vi "Class Reference FGV.vi"(7 "Options":T2, 8 "error in":errorcluster, 11 "Class Cluster In":T1) -> (0 "error out":errorcluster, 3 "Class Cluster Out":T1)   [LabVIEW 2023, in "HardwareAbstractionLayer_LVOOP.lvlib" / "Main.lvclass"]
uses:
  Main.lvclass
  Class Options.ctl
  Class Ref.ctl
  DMM/DMM.lvclass
  Function Generator/Function Generator.lvclass
  Oscilloscope/Oscilloscope.lvclass
  PowerSupply/PowerSupply.lvclass
  Teststand/Teststand.lvclass
  Analog Output/AO/AO.lvclass
  Analog Input/AI/AI.lvclass
  Database/Database.lvclass
  Digital Output/DO_class/DO.lvclass
  Digital Input/DI_class/DI.lvclass
  PWM Output/PWM Output_class/PWM Output.lvclass
  PWM Input/PWM Input_class/PWM Input.lvclass
  NI Switch/NISwitch_class/NISwitch.lvclass
  Modbus/Modbus_class/Modbus.lvclass
  CAN/CAN Lib/CAN_class/CAN.lvclass
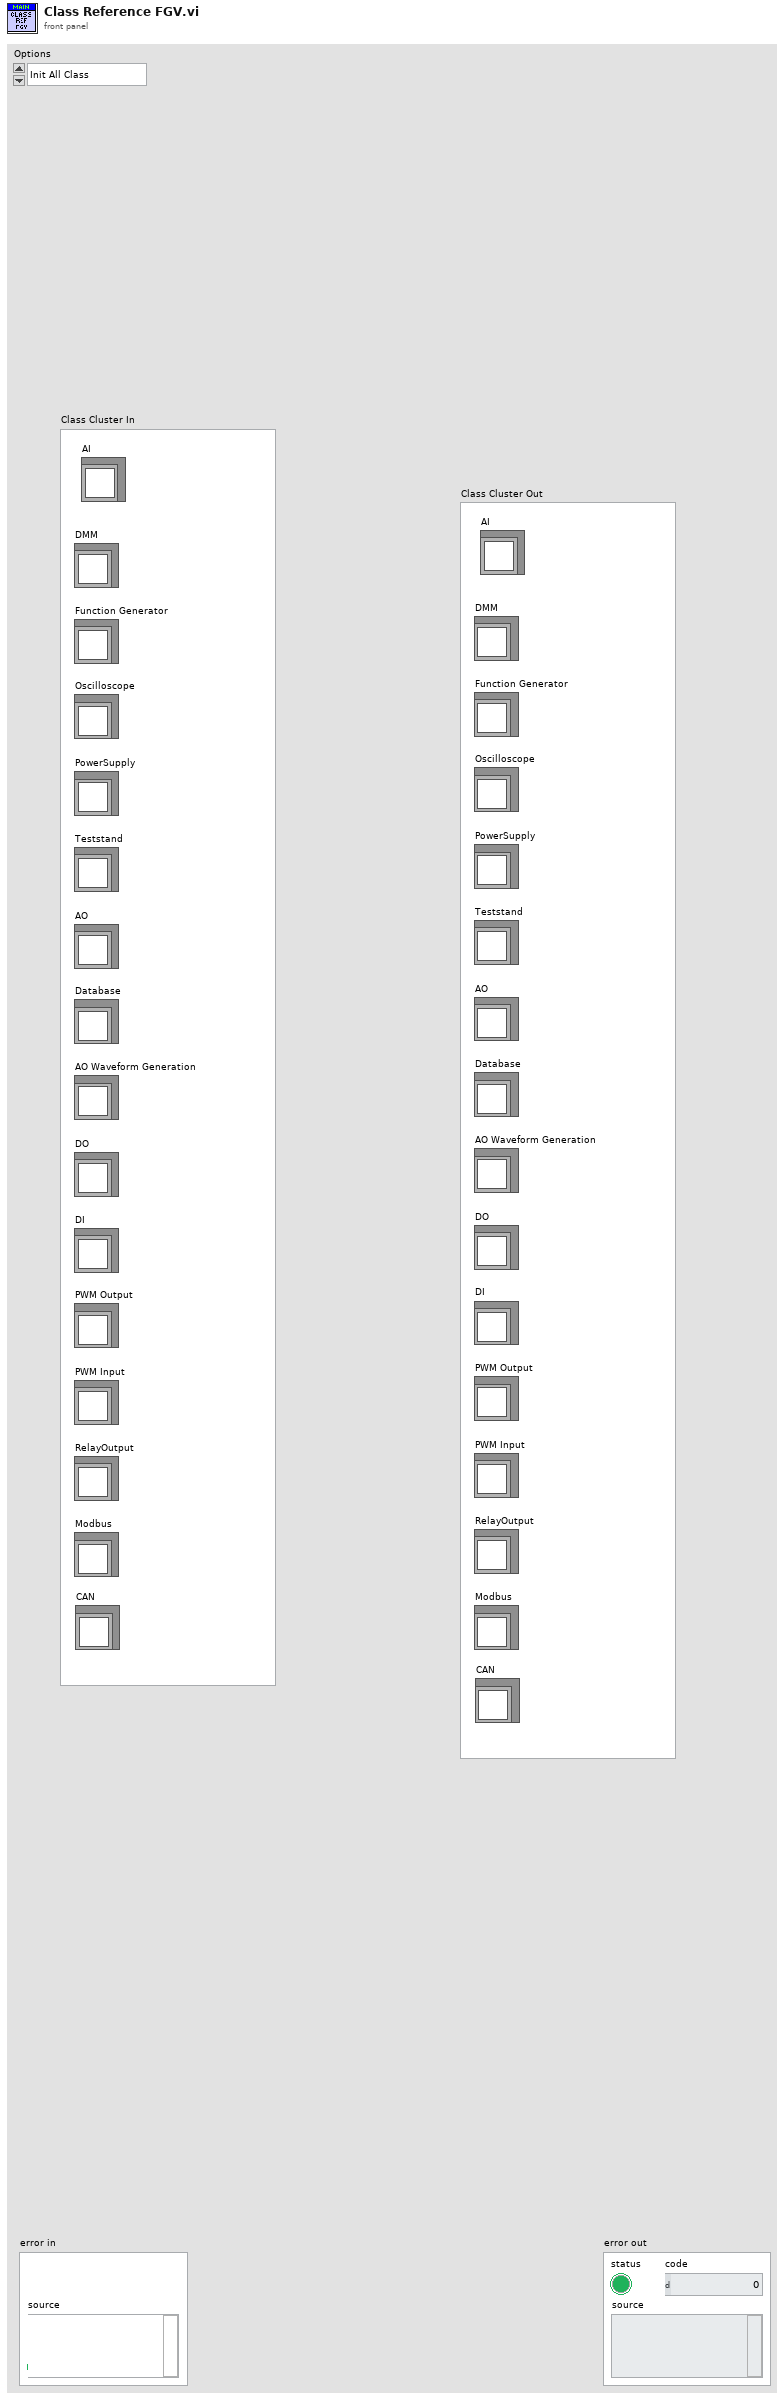
[diagram p1: front panel]
types:
  T1 = typedef "HardwareAbstractionLayer_LVOOP.lvlib/Main.lvclass/Class Ref.ctl" = cluster{"DMM":refnum<class "DMM.lvclass">, "Function Generator":refnum<class "Function Generator.lvclass">, "Oscilloscope":refnum<class "Oscilloscope.lvclass">, "PowerSupply":refnum<class "PowerSupply.lvclass">, "Teststand":refnum<class "Teststand.lvclass">, "AO":refnum<class "AO.lvclass">, "AI":refnum<class "AI.lvclass">, "Database":refnum<class "Database.lvclass">, "AO Waveform Generation":refnum<class "AO.lvclass">, "DO":refnum<class "DO.lvclass">, "DI":refnum<class "DI.lvclass">, "PWM Output":refnum<class "PWM Output.lvclass">, "PWM Input":refnum<class "PWM Input.lvclass">, "RelayOutput":refnum<class "NISwitch.lvclass">, "Modbus":refnum<class "Modbus.lvclass">, "CAN":refnum<class "CAN.lvclass">}
  T2 = typedef "HardwareAbstractionLayer_LVOOP.lvlib/Main.lvclass/Class Options.ctl" = enum16{"Init All Class", "Read All Class", "Write AI Class", "Write AO Class", "Write AO Waveform Generation", "Write DI Class", "Write DO Class", "Write PWM Input Class", "Write PWM Output Class", "Exit"}
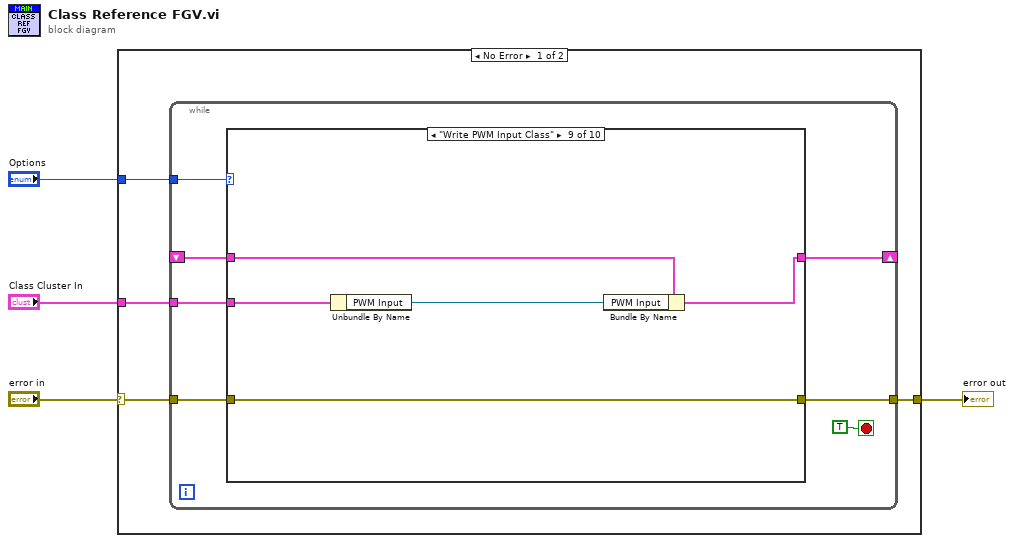
[diagram p0: block diagram]
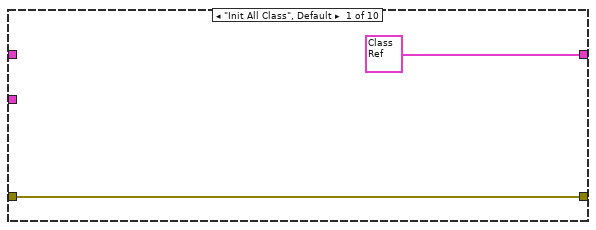
[diagram p2: hidden frame]
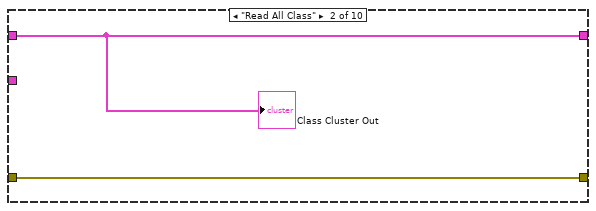
[diagram p3: hidden frame]
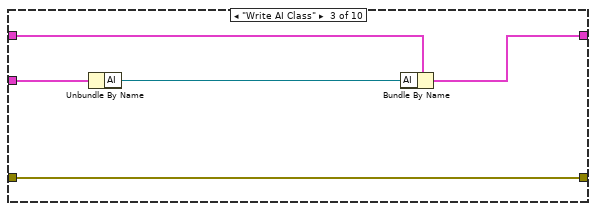
[diagram p4: hidden frame]
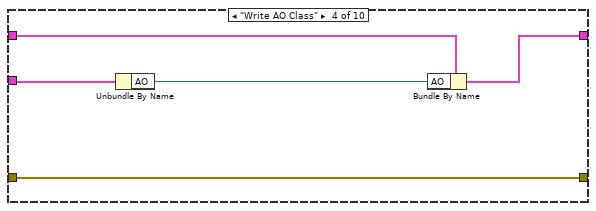
[diagram p5: hidden frame]
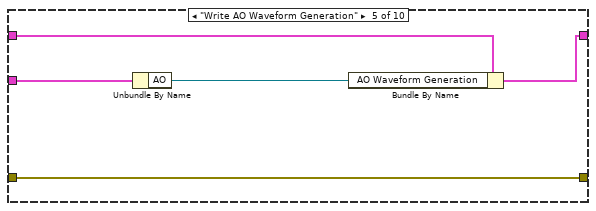
[diagram p6: hidden frame]
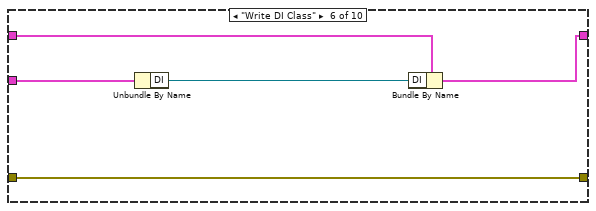
[diagram p7: hidden frame]
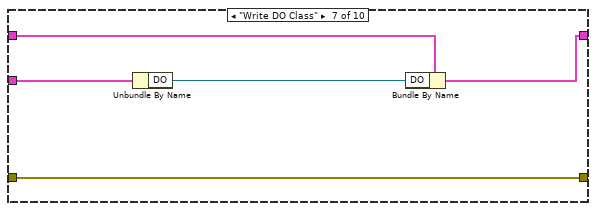
[diagram p8: hidden frame]
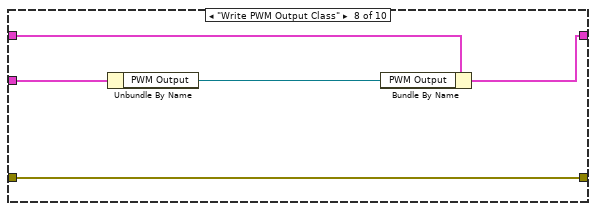
[diagram p9: hidden frame]
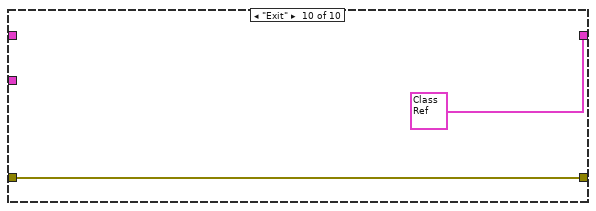
[diagram p10: hidden frame]
diagram:
  n1 = case shown="No Error" "error in" {
    selector: "error in" -> [w6 w57]
    tunnel: "Options" -> [w8 _]
    tunnel: "Class Cluster In" -> [w7 _]
    tunnel: [w5 w57] -> w1
    frame No Error {
      n2 = while {
        tunnel: w8 -> [w14]
        shift-right: [w12] -> _
        shift-left: _ -> [w13]
        tunnel: w7 -> [w11]
        tunnel: w6 -> [w10]
        tunnel: [w9] -> w5
        stop <- TRUE stop-if-true
        n3 = case shown="\"Write PWM Input Class\"" w14 {
          tunnel: w13 -> [_ w19 w23 w27 w32 w37 w42 w47 w52 _]
          tunnel: [T1 {"DMM"=refnum, "Function Generator"=refnum, "Oscilloscope"=refnum, "PowerSupply"=refnum, "Teststand"=refnum, "AO"=refnum, "AI"=refnum, "Database"=refnum, "AO Waveform Generation"=refnum, "DO"=refnum, "DI"=refnum, "PWM Output"=refnum, "PWM Input"=refnum, "RelayOutput"=refnum, "Modbus"=refnum, "CAN"=refnum} ("Class Cluster In") w19 w22 w26 w31 w36 w41 w46 w51 T1 {"DMM"=refnum, "Function Generator"=refnum, "Oscilloscope"=refnum, "PowerSupply"=refnum, "Teststand"=refnum, "AO"=refnum, "AI"=refnum, "Database"=refnum, "AO Waveform Generation"=refnum, "DO"=refnum, "DI"=refnum, "PWM Output"=refnum, "PWM Input"=refnum, "RelayOutput"=refnum, "Modbus"=refnum, "CAN"=refnum} ("Class Cluster In")] -> w12
          tunnel: w11 -> [_ _ w21 w25 w30 w35 w40 w45 w50 _]
          tunnel: w10 -> [w16 w18 w24 w29 w34 w39 w44 w49 w54 w55]
          tunnel: [w16 w18 w24 w29 w34 w39 w44 w49 w54 w55] -> w9
          frame "Init All Class", Default {
          }
          frame "Read All Class" {
            "Class Cluster Out" <- w19
          }
          frame "Write AI Class" {
            n4 = Unbundle By Name(w21) -> ("AI"=w20:refnum<class "AI.lvclass">)
            n5 = Bundle By Name(cluster=w23, "AI"=w20) -> (w22:T1)
          }
          frame "Write AO Class" {
            n6 = Unbundle By Name(w25) -> ("AO"=w28:refnum<class "AO.lvclass">)
            n7 = Bundle By Name(cluster=w27, "AO"=w28) -> (w26:T1)
          }
          frame "Write AO Waveform Generation" {
            n8 = Unbundle By Name(w30) -> ("AO"=w33:refnum<class "AO.lvclass">)
            n9 = Bundle By Name(cluster=w32, "AO Waveform Generation"=w33) -> (w31:T1)
          }
          frame "Write DI Class" {
            n10 = Unbundle By Name(w35) -> ("DI"=w38:refnum<class "DI.lvclass">)
            n11 = Bundle By Name(cluster=w37, "DI"=w38) -> (w36:T1)
          }
          frame "Write DO Class" {
            n12 = Unbundle By Name(w40) -> ("DO"=w43:refnum<class "DO.lvclass">)
            n13 = Bundle By Name(cluster=w42, "DO"=w43) -> (w41:T1)
          }
          frame "Write PWM Output Class" {
            n14 = Unbundle By Name(w45) -> ("PWM Output"=w48:refnum<class "PWM Output.lvclass">)
            n15 = Bundle By Name(cluster=w47, "PWM Output"=w48) -> (w46:T1)
          }
          frame "Write PWM Input Class" {
            n16 = Unbundle By Name(w50) -> ("PWM Input"=w53:refnum<class "PWM Input.lvclass">)
            n17 = Bundle By Name(cluster=w52, "PWM Input"=w53) -> (w51:T1)
          }
          frame "Exit" {
          }
        }
      }
    }
    frame Error {
    }
  }
  "error out" <- w1
